vi "Get CYMG Shift.vi"(8 "error in (no error)":errorcluster, 10 "iYShift":i32, 11 "iXshift":i32) -> (0 "error out":errorcluster, 1 "function return":u32, 2 "iYShift out":i32, 3 "iXshift out":i32)   [LabVIEW 2014, in "atmcd32d.lvlib"]
doc: "unsigned int WINAPI GetCYMGShift(int * iXshift, int * iYShift);"
uses:
  atmcd32d.lvlib
  atmcd32d.dll
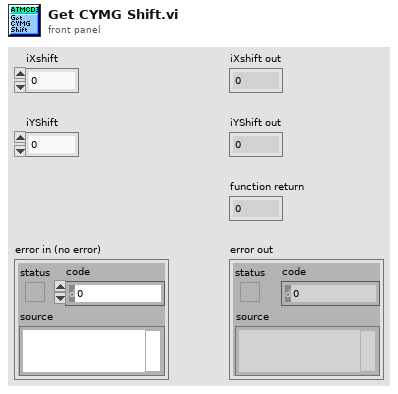
[diagram p1: front panel]
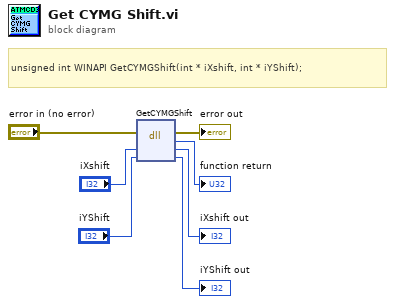
[diagram p0: block diagram]
diagram:
  # "unsigned int WINAPI GetCYMGShift(int * iXshift, int * iYShift);"
  n1 = dll-call lib="C:/Users/Bakir/Documents/Lambda2-Testing/lib/Andorlib/atmcd32d.*" fn="GetCYMGShift"(error in="error in (no error)", "iXshift"="iXshift", "iYShift"="iYShift") -> (error out=→"error out":errorcluster, →"function return":u32, "iXshift"=→"iXshift out":i32, "iYShift"=→"iYShift out":i32)  [unwired: 2 in, 1 out]
